vi "Sample Rate Write.vi"(4 "error in (no error)":errorcluster, 5 "Value":dbl=51200.0, 6 "Container State":T2, 7 "Display State In":T1) -> (0 "error out":errorcluster, 3 "Display State Out":T1)   [LabVIEW 2017, in "Test Signal Configuration.xctl"]
uses:
  <vilib>/addons/_XControls/Function Generator Configuration/Test Signal Configuration.xctl
  <vilib>/_xctls/Container State.ctl
  <vilib>/addons/_XControls/Function Generator Configuration/Controls/State.ctl
  <vilib>/_xctls/XControlSupport.lvlib
panel:
  # "Replace the Value Control below with a Control of desired type.\nDo not remove this Control or the others from the connector pane.\nDo not change the connector pane pattern.\nThe Value control should always be the third terminal from top on the input side in the connector pane."
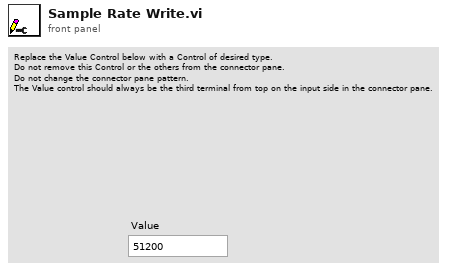
[diagram p1: front panel]
types:
  T1 = typedef "Test Signal Configuration.xctl/State.ctl" = cluster{"Attributes":variant}
  T2 = typedef "XControlSupport.lvlib/Container State.ctl" = cluster{"Indicator?":bool, "Run Mode?":bool, " Refnum":refnum<vi>}
  T3 = typedef "Test Signal Configuration.xctl/signal type.ctl" = enum32{"None", "Tone", "Multitone", "Discrete Sweep", "Continuous Sweep", "Noise"}
  T4 = cluster{"Signal":cluster{"Sample Rate":cluster{"name":string, "default":dbl}, "Signal Type":cluster{"name":string, "signal type":T3}, "Amplitude":cluster{"name":string, "default":dbl}, "Offset":cluster{"name":string, "default":dbl}}, "Function":cluster{"Info":cluster{"name":string, "default":variant}, "Type":cluster{"name":string, "default":u16}, "Frequency":cluster{"name":string, "default":dbl}, "Phase":cluster{"name":string, "default":dbl}}, "Continuous Sweep":cluster{"Info":cluster{"name":string, "default":variant}, "Start":cluster{"name":string, "default":dbl}, "Stop":cluster{"name":string, "default":dbl}, "Duration":cluster{"name":string, "default":dbl}, "Profile":cluster{"name":string, "default":enum16{"Linear", "Logarithmic"}}}, "Discrete Sweep":cluster{"Info":cluster{"name":string, "default":variant}, "Start":cluster{"name":string, "default":dbl}, "Stop":cluster{"name":string, "default":dbl}, "Cycles":cluster{"name":string, "default":dbl}, "Time":cluster{"name":string, "default":dbl}, "Spacing":cluster{"name":string, "default":enum16{"Linear", "Logarithmic"}}, "Steps":cluster{"name":string, "default":i32}}, "Multitone":cluster{"Info":cluster{"name":string, "multitone info":cluster{"frequency":dbl, "amplitude":dbl, "phase":dbl}[]}}, "Noise":cluster{"Info":cluster{"name":string, "default":variant}, "Type":cluster{"name":string, "default":u16}, "Amplitude PDF":cluster{"name":string, "default":enum16{"Gaussian", "Rectangular", "Triangular"}}, "Level":cluster{"name":string, "default":dbl}, "Seed":cluster{"name":string, "default":i32}}, "Configuration":cluster{"Min Frequency":cluster{"name":string, "default":dbl}, "Max Frequency":cluster{"name":string, "default":dbl}, "Max Amplitude":cluster{"name":string, "default":dbl}}}
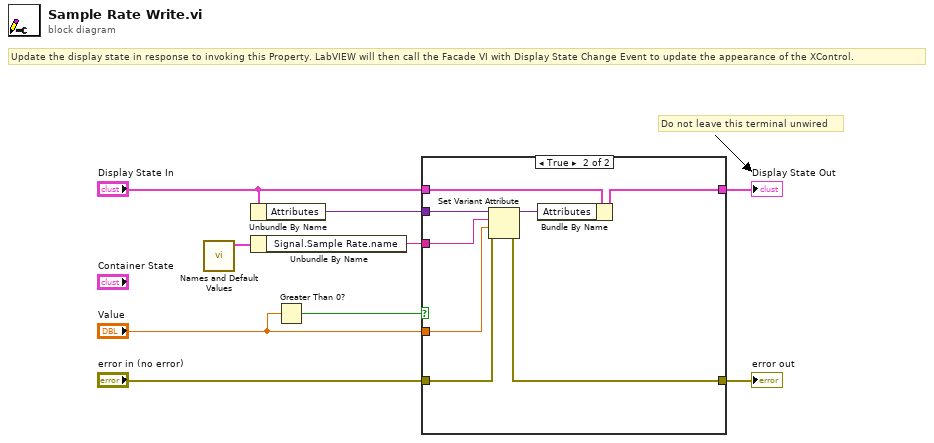
[diagram p0: block diagram]
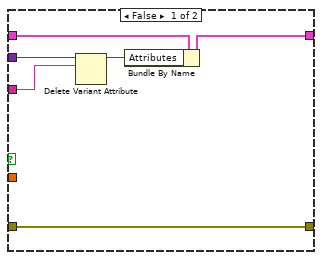
[diagram p2: hidden frame]
diagram:
  # "Do not leave this terminal unwired"
  # "Update the display state in response to invoking this Property. LabVIEW will then call the Facade VI with Display State Change Event to update the appearance of the XControl."
  n1 = call <vilib>:"Names and Default Values.vi"() -> ("Names and Default Values"=w9:T4)  [unwired: 11 in]
  n2 = Unbundle By Name("Display State In") -> ("Attributes"=w8:variant)
  n3 = Unbundle By Name(w9) -> ("Signal.Sample Rate.name"=w7:string)
  n4 = Greater Than 0?(x="Value") -> (x > 0?=w3:bool)
  n5 = case shown="True" w3 {
    tunnel: w8 -> [w14 w23]
    tunnel: w7 -> [w11 w22]
    tunnel: "Display State In" -> [w13 w21]
    tunnel: [w12 w20] -> w5
    tunnel: "Value" -> [_ w18]
    tunnel: "error in (no error)" -> [w10 w17]
    tunnel: [w10 w16] -> w1
    frame False {
      n6 = Delete Variant Attribute(6:w11, 7:w14) -> (3:w15:variant)  [unwired: 1 in, 2 out]
      n7 = Bundle By Name(cluster=w13, "Attributes"=w15) -> (w12:T1)
    }
    frame True {
      n8 = Set Variant Attribute(Variant=w23, name=w22, value=w18, error in=w17) -> (Variant out=w19:variant, error out=w16:errorcluster)  [unwired: 1 out]
      n9 = Bundle By Name(cluster=w21, "Attributes"=w19) -> (w20:T1)
    }
  }
  "error out" <- w1
  "Display State Out" <- w5
